vi "GetPixelColor.vi"(8 "错误输入":errorcluster, 10 "Coords":T1, 11 "HDC":u32) -> (0 "错误输出":errorcluster, 3 "Color":u32(colorbox) caption="颜色")   [LabVIEW 2018, in "Win32API.lvlib"]
uses:
  <vilib>/Utility/miscctls.llb/LVPoint32TypeDef.ctl
  Win32API.lvlib
  Gdi32.dll
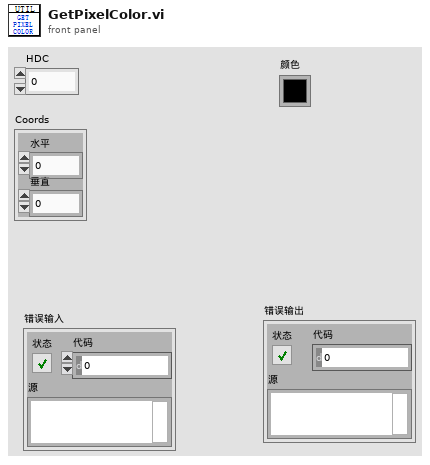
[diagram p1: front panel]
types:
  T1 = typedef "LVPoint32TypeDef.ctl" = cluster{"Horizontal":i32, "Vertical":i32}
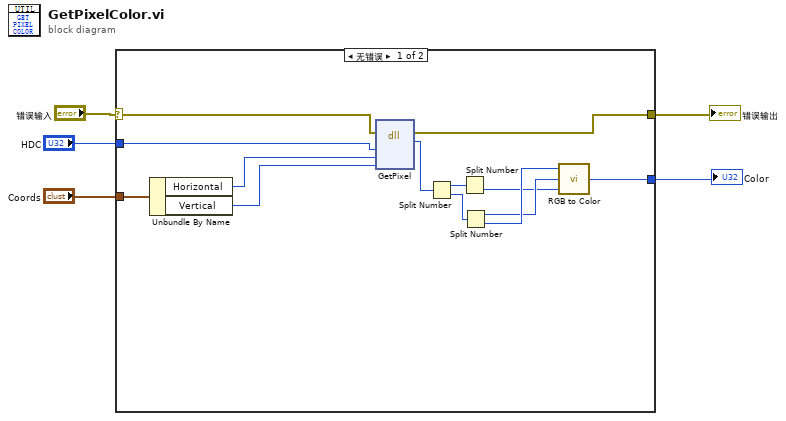
[diagram p0: block diagram]
diagram:
  n1 = case shown="无错误" "错误输入" {
    selector: "错误输入" -> [w9 w19]
    tunnel: [w13 w19] -> w5
    tunnel: "Coords" -> [w8 _]
    tunnel: "HDC" -> [w7 _]
    tunnel: [w6 _] -> w1
    frame No Error {
      n2 = Unbundle By Name(w8) -> ("Horizontal"=w14:i32, "Vertical"=w15:i32)
      n3 = dll-call lib="Gdi32.dll" fn="GetPixel"(error in=w9, "Handle Context"=w7, "x"=w14, "y"=w15) -> (error out=w13:errorcluster, "Color"=w18:u32)  [unwired: 5 in, 1 out]
      n4 = Split Number(x=w18) -> (hi(x)=w17:u16, lo(x)=w16:u16)
      n5 = Split Number(x=w17) -> (lo(x)=w10:u8)  [unwired: 1 out]
      n6 = Split Number(x=w16) -> (hi(x)=w11:u8, lo(x)=w12:u8)
      n7 = call <vilib>:"RGB to Color.vi"("B"=w10, "G"=w11, "R"=w12) -> ("Color"=w6:u32)
    }
    frame Error {
    }
  }
  "错误输出" <- w5
  "Color" <- w1
